vi "Database-CheckExist.vi"(8 "error in":errorcluster, 9 "Serial":string, 10 "Ref":string) -> (0 "error out":errorcluster)   [LabVIEW 2016]
doc: "Go to DB->WriteStationValues action\nReturn boolean flag to show if data was saved to DB successfully\n\nWabco 2017 All right reserved\nAuthor: maciej.szupienko@wabco-auto.com"
uses:
  Database.Action.ctl
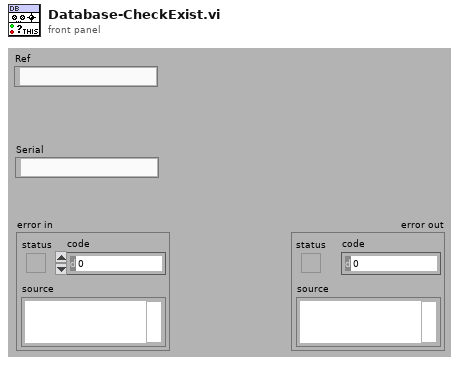
[diagram p1: front panel]
types:
  T1 = typedef "Database.Action.ctl" = enum32{"idle", "constructor", "destructor", "--- DB ---", "Setup", "Disconnect", "Connect", "GetThisStatus"}
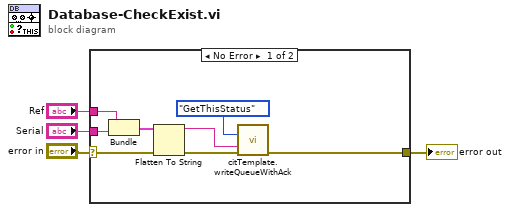
[diagram p0: block diagram]
diagram:
  n1 = case shown="No Error" "error in" {
    selector: "error in" -> [w12 w13]
    tunnel: [w5 w13] -> w3
    tunnel: "Serial" -> [w9 _]
    tunnel: "Ref" -> [w8 _]
    frame No Error {
      n2 = Bundle("Ref"=w8, "Serial"=w9) -> (w10:cluster{"Ref":string, "Serial":string})  [unwired: 1 in]
      n3 = Flatten To String(anything=w10, error in (no error)=w12) -> (data string=w6:string, error out=w11:errorcluster)  [unwired: 2 in, 1 out]
      n4 = call "citTemplate.writeQueueWithAck.vi"("event in"=Database.Action."GetThisStatus" ("Action"), "(flatten) data in"=w6, "error in (no error)"=w11) -> ("error out"=w5:errorcluster)  [unwired: 10 in, 2 out]
    }
    frame Error {
    }
  }
  "error out" <- w3
